vi "Configure Trigger Characteristics.vi"(0 "VISA resource name":refnum<visa-resource-name>, 1 "Enable High Frequency Filter (F: Disable)":bool, 2 "Trigger Level Source (0: Channel 1)":i32(ring) items=["Channel 1", "Channel 2", "Channel 3", "Channel 4"], 3 "Low Trigger Voltage Level (1 V)":dbl=1.0, 5 "Trigger Type (0: Edge)":i32(ring) items=["Edge", "Glitch", "Pattern", "TV", "Edge Burst", "Runt", "Setup Hold", "Transition", "Serial Bus 1", "Serial Bus 2", "USB", "Delay", "Or"], 7 "Holdoff Time (4E-8 S)":dbl=4e-08, 9 "Trigger Sweep (0: Auto)":i32(ring) items=["Auto", "Normal"], 11 "error in (no error)":errorcluster, 12 "Enable Noise Filter (F: Disable)":bool, 13 "High Trigger Voltage Level (1 V)":dbl=1.0) -> (4 "VISA resource name out":refnum<visa-resource-name>, 15 "error out":errorcluster)   [LabVIEW 2015, in "Agilent 2000 3000 X-Series.lvlib"]
doc: "Configures the basic settings of trigger. Note that these characteristics act on the currently selected source, so before calling this VI ensure tat the proper source has been selected. Do this by calling <b>Configure Trigger </b> VI."
uses:
  <instrlib>/Agilent 2000 3000 X-Series/Agilent 2000 3000 X-Series.lvlib
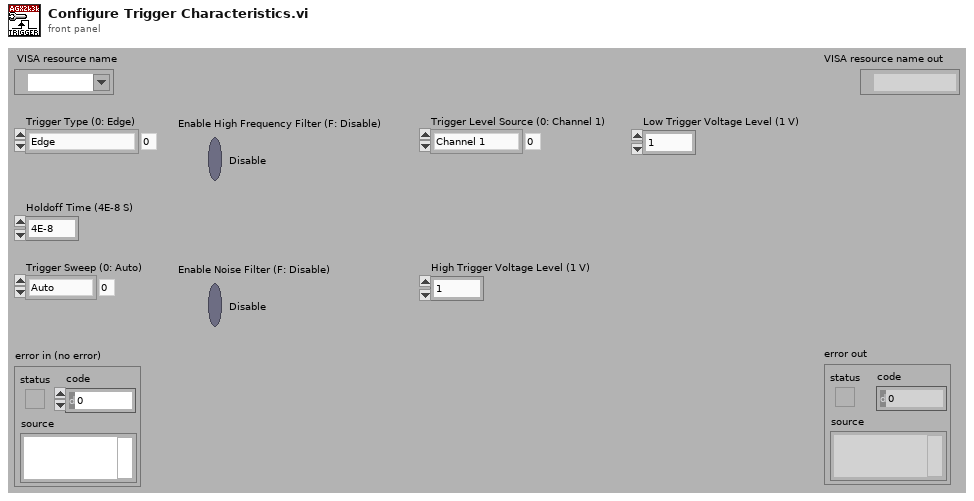
[diagram p1: front panel]
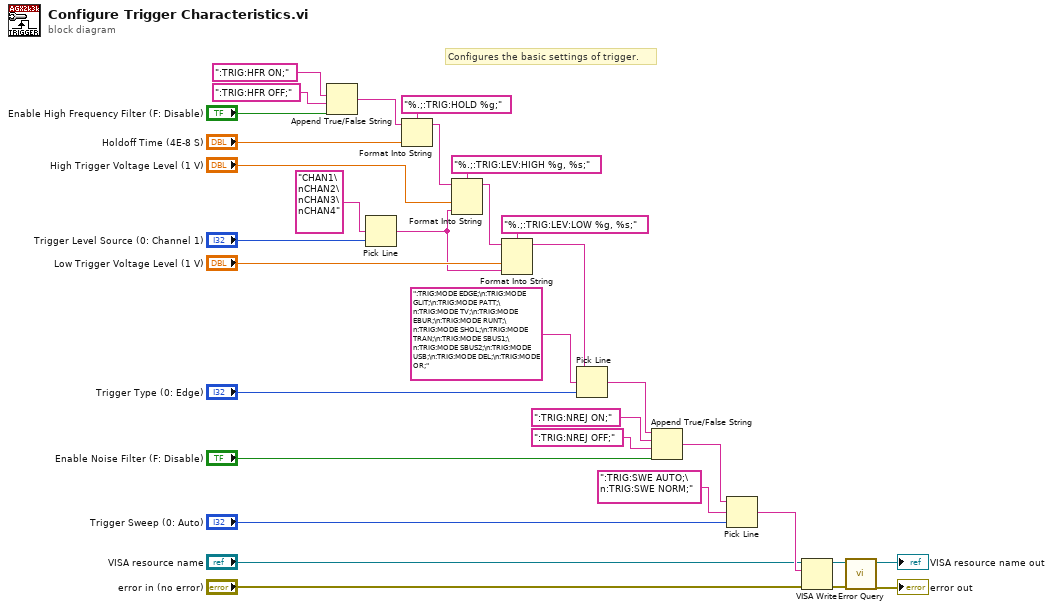
[diagram p0: block diagram]
diagram:
  # "Configures the basic settings of trigger."
  n1 = Append True/False String(1:"Enable High Frequency Filter (F: Disable)", 2:":TRIG:HFR OFF;", 3:":TRIG:HFR ON;") -> (0:w29:string)  [unwired: 1 out]
  n2 = Pick Line(multi-line string="CHAN1\nCHAN2\nCHAN3\nCHAN4", line index="Trigger Level Source (0: Channel 1)") -> (output string=w1:string)  [unwired: 1 out]
  n3 = Format Into String(format string="%.;:TRIG:HOLD %g;", initial string=w29, "Holdoff Time (4E-8 S)") -> (resulting string=w26:string)  [unwired: 1 in, 1 out]
  n4 = Format Into String(format string="%.;:TRIG:LEV:HIGH %g, %s;", initial string=w26, "High Trigger Voltage Level (1 V)", w1) -> (resulting string=w23:string)  [unwired: 1 in, 1 out]
  n5 = Format Into String(format string="%.;:TRIG:LEV:LOW %g, %s;", initial string=w23, "Low Trigger Voltage Level (1 V)", w1) -> (resulting string=w18:string)  [unwired: 1 in, 1 out]
  n6 = Pick Line(string ("")=w18, multi-line string=":TRIG:MODE EDGE;\n:TRIG:MODE GLIT;\n:TRIG:MODE PATT;\n:TRIG:MODE TV;\n:TRIG:MODE EBUR;\n:TRIG:MODE RUNT;\n:TRIG:MODE SHOL;\n:TRIG:MODE TRAN;\n:TRIG:MODE SBUS1;\n:TRIG:MODE SBUS2;\n:TRIG:MODE USB;\n:TRIG:MODE DEL;\n:TRIG:MODE OR;", line index="Trigger Type (0: Edge)") -> (output string=w17:string)
  n7 = Append True/False String(1:"Enable Noise Filter (F: Disable)", 2:":TRIG:NREJ OFF;", 3:":TRIG:NREJ ON;", 4:w17) -> (0:w11:string)
  n8 = Pick Line(string ("")=w11, multi-line string=":TRIG:SWE AUTO;\n:TRIG:SWE NORM;", line index="Trigger Sweep (0: Auto)") -> (output string=w10:string)
  n9 = VISA Write(VISA resource name="VISA resource name", write buffer=w10, error in (no error)="error in (no error)") -> (VISA resource name out=w7:refnum<visa-resource-name>, error out=w6:errorcluster)  [unwired: 1 out]
  n10 = call <instrlib>:"Error Query.vi"("error in (no error)"=w6, "VISA resource name"=w7) -> ("error out"=→"error out":errorcluster, "VISA resource name out"=→"VISA resource name out":refnum<visa-resource-name>)  [unwired: 8 out]
